vi "Calculate New Analysis Start And End Angle.vi"(8 "Right Wing?":bool, 9 "End Angle":fxp<+/-,17,2>, 10 "Start Angle":fxp<+/-,17,2>, 11 "Sector":u8) -> (2 "Start Angle Out":fxp<+/-,17,2>, 3 "End Angle Out":fxp<+/-,17,2>)   [LabVIEW 2013]
uses:
  <vilib>/rvi/Analysis/common/FxpNativeNode/niFpgaFxpNative.xnode
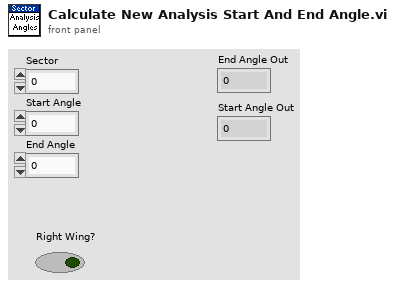
[diagram p1: front panel]
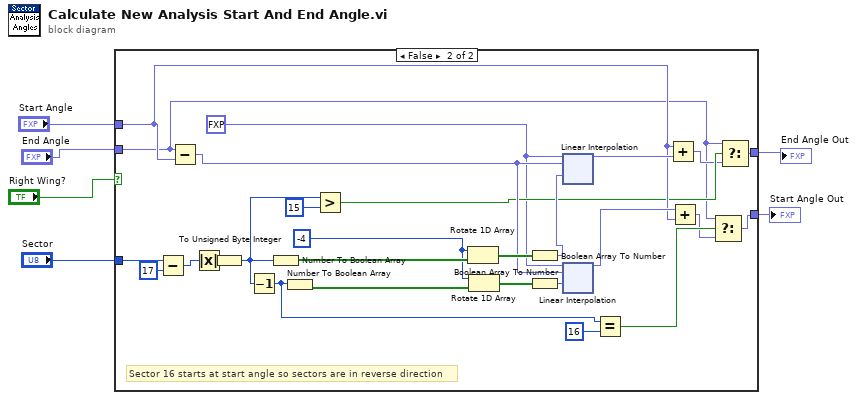
[diagram p0: block diagram]
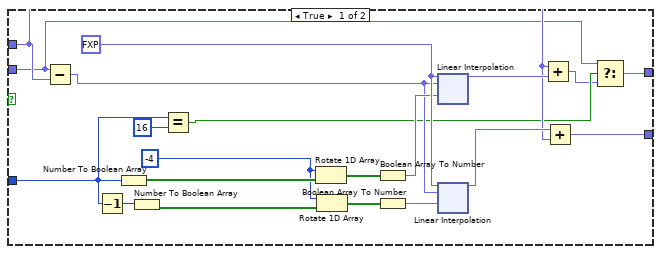
[diagram p2: hidden frame]
diagram:
  n1 = case shown="False" "Right Wing?" {
    tunnel: "Start Angle" -> [w14 w65]
    tunnel: [w13 w50] -> w5
    tunnel: "Sector" -> [w12 w64]
    tunnel: [w8 w60] -> w3
    tunnel: "End Angle" -> [w7 w49]
    frame True {
      w22 = -4 ("n")
      w18 = fxp<+/-,17,2> 0.0 ("Start Angle")
      n2 = Subtract(x=w7, y=w14) -> (x-y=w16:fxp<+/-,18,2>)
      n3 = Decrement(x=w12) -> (x-1=w23:u8)
      n4 = Number To Boolean Array(number=w12) -> (Boolean array=w25:bool[])
      n5 = Number To Boolean Array(number=w23) -> (Boolean array=w21:bool[])
      n6 = Equal?(x=w12, y=u8 16) -> (x = y?=w10:bool)
      n7 = Rotate 1D Array(1:w25, 2:w22) -> (0:w24:bool[])
      n8 = Rotate 1D Array(1:w21, 2:w22) -> (0:w20:bool[])
      n9 = Boolean Array To Number(Boolean array=w24) -> (number=w17:fxp<+,8,0>)
      n10 = Boolean Array To Number(Boolean array=w20) -> (number=w19:fxp<+,8,0>)
      n11 = xnode ("Linear Interpolation")("y0"=w18, "y1"=w16, "x"=w17) -> ("y"=w26:fxp<+/-,17,2>)
      n12 = xnode ("Linear Interpolation")("y0"=w18, "y1"=w16, "x"=w19) -> ("y"=w15:fxp<+/-,17,2>)
      n13 = Add(x=w14, y=w26) -> (x+y=w9:fxp<+/-,17,2>)
      n14 = Add(x=w15, y=w14) -> (x+y=w13:fxp<+/-,17,2>)
      n15 = Select(t=w7, s=w10, f=w9) -> (s? t:f=w8:fxp<+/-,17,2>)
    }
    frame False {
      w72 = -4 ("n")
      w55 = fxp<+/-,17,2> 0.0 ("Start Angle")
      # "Sector 16 starts at start angle so sectors are in reverse direction"
      n16 = Subtract(x=w64, y=i16 17) -> (x-y=w57:i16)
      n17 = Subtract(x=w49, y=w65) -> (x-y=w67:fxp<+/-,18,2>)
      n18 = Absolute Value(x=w57) -> (abs(x)=w58:i16)
      n19 = To Unsigned Byte Integer(number=w58) -> (unsigned 8bit integer=w56:u8)
      n20 = Decrement(x=w56) -> (x-1=w53:u8)
      n21 = Number To Boolean Array(number=w56) -> (Boolean array=w74:bool[])
      n22 = Number To Boolean Array(number=w53) -> (Boolean array=w71:bool[])
      n23 = Greater?(x=w56, y=u8 15) -> (0:w62:bool)
      n24 = Rotate 1D Array(1:w74, 2:w72) -> (0:w73:bool[])
      n25 = Rotate 1D Array(1:w71, 2:w72) -> (0:w70:bool[])
      n26 = Boolean Array To Number(Boolean array=w73) -> (number=w68:fxp<+,8,0>)
      n27 = Boolean Array To Number(Boolean array=w70) -> (number=w69:fxp<+,8,0>)
      n28 = xnode ("Linear Interpolation")("y0"=w55, "y1"=w67, "x"=w68) -> ("y"=w75:fxp<+/-,17,2>)
      n29 = xnode ("Linear Interpolation")("y0"=w55, "y1"=w67, "x"=w69) -> ("y"=w66:fxp<+/-,17,2>)
      n30 = Equal?(x=w53, y=u8 16) -> (x = y?=w52:bool)
      n31 = Add(x=w65, y=w75) -> (x+y=w61:fxp<+/-,17,2>)
      n32 = Add(x=w66, y=w65) -> (x+y=w51:fxp<+/-,17,2>)
      n33 = Select(t=w49, s=w52, f=w51) -> (s? t:f=w50:fxp<+/-,17,2>)
      n34 = Select(t=w49, s=w62, f=w61) -> (s? t:f=w60:fxp<+/-,17,2>)
    }
  }
  "End Angle Out" <- w3
  "Start Angle Out" <- w5
